vi "speed_test.vi"() -> ()   [LabVIEW 2010]
panel:
  out "XY Graph 2":cluster{i32[], dbl[]}(graph)
  out "Numeric":i32
  out "XY Graph":cluster{i32[], dbl[]}(graph)
  out "resulting string":string
  in  "spot":dbl[](array[numeric])
  # "x"
  # "y"
  # "z"
  # "I"
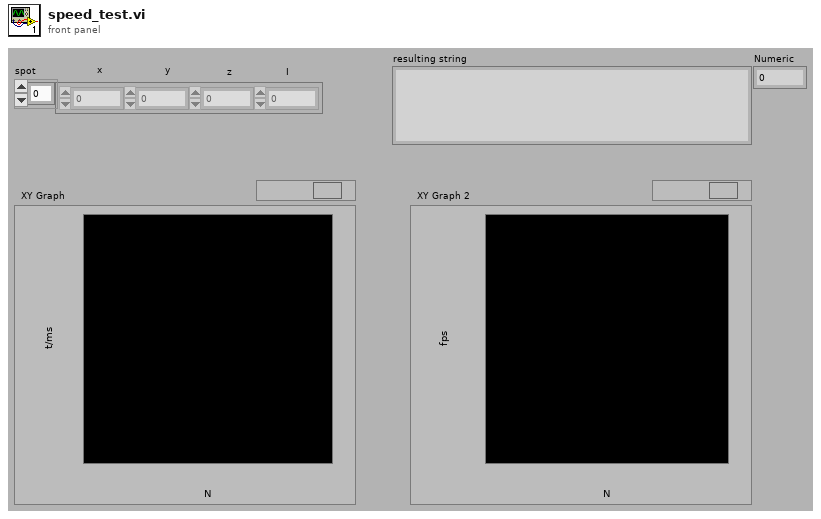
[diagram p1: front panel]
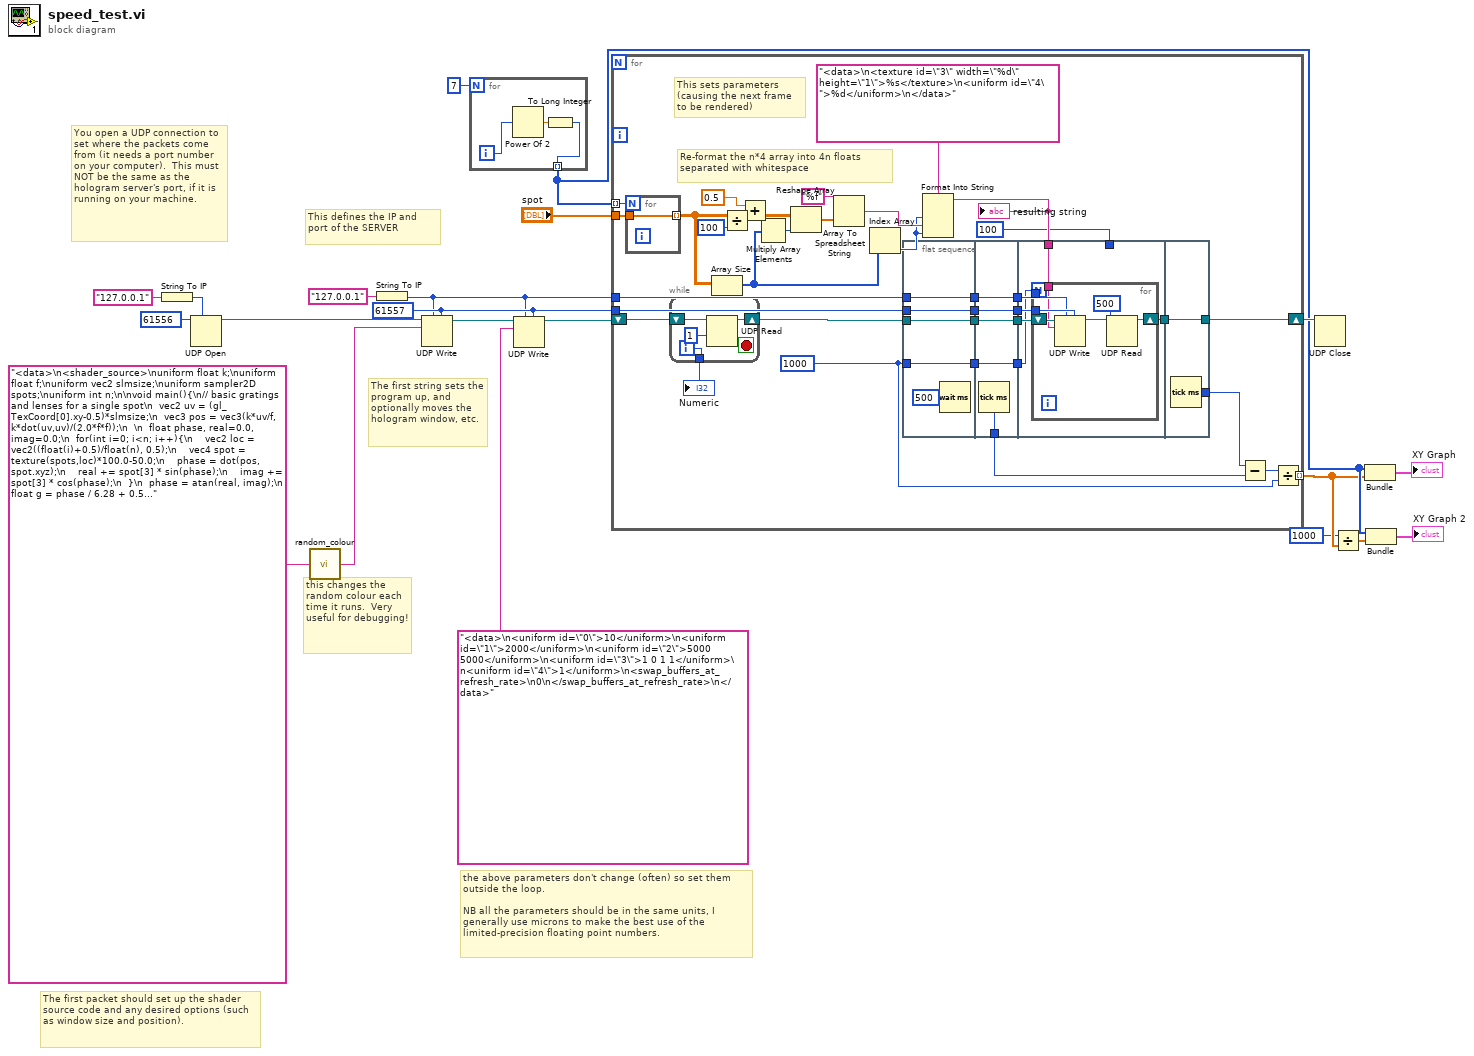
[diagram p0: block diagram]
diagram:
  w15 = u16 61557 ("port")
  # "The first packet should set up the shader source code and any desired options (such as window size and position)."
  # "This defines the IP and port of the SERVER"
  # "the above parameters don't change (often) so set them outside the loop.\n\nNB all the parameters should be in the same units, I generally use microns to make the best use of the limited-precision floating point numbers."
  # "You open a UDP connection to set where the packets come from (it needs a port number on your computer).  This must NOT be the same as the hologram server's port, if it is running on your machine."
  # "The first string sets the program up, and optionally moves the hologram window, etc."
  # "this changes the random colour each time it runs.  Very useful for debugging!"
  n1 = String To IP(1:"127.0.0.1" ("name")) -> (0:w14:u32)
  n2 = UDP Open(7:w14, 11:u16 61556 ("port")) -> (port=w21:refnum<k16>)  [unwired: 3 in, 2 out]
  n3 = call "random_colour.vi"("string in"="<data>\n<shader_source>\nuniform float k;\nuniform float f;\nuniform vec2 slmsize;\nuniform sampler2D spots;\nuniform int n;\n\nvoid main(){\n// basic gratings and lenses for a single spot\n  vec2 uv = (gl_TexCoord[0].xy-0.5)*slmsize;\n  vec3 pos = vec3(k*uv/f, k*dot(uv,uv)/(2.0*f*f));\n  \n  float phase, real=0.0, imag=0.0;\n  for(int i=0; i<n; i++){\n    vec2 loc = vec2((float(i)+0.5)/float(n), 0.5);\n    vec4 spot = texture(spots,loc)*100.0-50.0;\n    phase = dot(pos, spot.xyz);\n    real += spot[3] * sin(phase);\n    imag += spot[3] * cos(phase);\n  }\n  phase = atan(real, imag);\n  float g = phase / 6.28 + 0.5; // map -pi to pi onto zero to one\n\n  gl_FragColor=vec4(g,g,g,1.0);\n\n//  gl_FragColor = vec4(%%randcol%%);\n}\n</shader_source>\n<window_rect>\n0 0 512 512\n</window_rect>\n<network_reply>\n1\n</network_reply>\n</data> " ("data in")) -> ("string out, with %%randcol%% replaced with a 4-element colour"=w16:string)
  n4 = String To IP(1:"127.0.0.1" ("name")) -> (0:w9:u32)
  n5 = UDP Write(address=w9, port or service name=w15, connection ID=w21, data in=w16) -> (3:w12:refnum<k16>)  [unwired: 2 in, 1 out]
  n6 = for {
    N: 7 -> [_]
    tunnel: [w22] -> w4 mode=indexing
    i -> [w24]
    n7 = Power Of 2(x=w24) -> (2^x=w23:dbl)
    n8 = To Long Integer(number=w23) -> (32bit integer=w22:i32)
  }
  n9 = UDP Write(address=w9, port or service name=w15, connection ID=w12, data in="<data>\n<uniform id=\"0\">10</uniform>\n<uniform id=\"1\">2000</uniform>\n<uniform id=\"2\">5000 5000</uniform>\n<uniform id=\"3\">1 0 1 1</uniform>\n<uniform id=\"4\">1</uniform>\n<swap_buffers_at_refresh_rate>\n0\n</swap_buffers_at_refresh_rate>\n</data>") -> (3:w13:refnum<k16>)  [unwired: 2 in, 1 out]
  n10 = for {
    tunnel: w15 -> [w50]
    tunnel: w9 -> [w48]
    tunnel: [w30] -> w2 mode=indexing
    tunnel: "spot" -> [w29]
    shift-right: [w51] -> w19
    shift-left: w13 -> [w49]
    tunnel: w4 -> [w27] mode=indexing
    w31 = 1000
    # "Re-format the n*4 array into 4n floats separated with whitespace"
    # "This sets parameters\n(causing the next frame\nto be rendered)"
    n11 = for {
      N: w27 -> [_]
      tunnel: w29 -> [w66]
      tunnel: [w66] -> w28 mode=indexing
    }
    n12 = while {
      shift-right: [w64] -> w26
      shift-left: w49 -> [w65]
      tunnel: [w62] -> w25
      i -> [w62]
      stop <- w61 stop-if-true
      n13 = UDP Read(connection ID=w65, timeout ms (25000)=1) -> (error out=w61:errorcluster, 3:w64:refnum<k16>)  [unwired: 2 in, 3 out]
    }
    "Numeric" <- w25
    n14 = Array Size(array=w28) -> (size(s)=w45:i32[])
    n15 = Divide(x=w28, y=100) -> (x/y=w39:dbl[][])
    n16 = Add(x=0.5, y=w39) -> (x+y=w37:dbl[][])
    n17 = Multiply Array Elements(1:w45) -> (0:w44:i32)
    n18 = Reshape Array(w37, w44) -> (w43:dbl[])
    n19 = Array To Spreadsheet String(array=w43, 3:"%f" ("format string")) -> (spreadsheet string=w42:string)  [unwired: 1 in]
    n20 = Index Array(array=w45) -> (element=w35:i32)  [unwired: 1 in]
    n21 = flat-sequence {
      tunnel: w31 -> [w68]
      tunnel: w48 -> [w69]
      tunnel: w26 -> [w70]
      tunnel: w50 -> [w71]
      tunnel: [w71] -> w60
      tunnel: [w70] -> w59
      tunnel: [w69] -> w58
      tunnel: [w68] -> w57
      tunnel: [w76] -> w56
      tunnel: [w75] -> w55
      tunnel: [w74] -> w54
      tunnel: [w73] -> w53
      tunnel: w60 -> [w76]
      tunnel: w59 -> [w75]
      tunnel: w58 -> [w74]
      tunnel: w57 -> [w73]
      tunnel: [w72] -> w33
      tunnel: w47 -> [w78]
      tunnel: u32 100 ("millisecond multiple") -> [_]
      tunnel: w56 -> [w81]
      tunnel: w55 -> [w80]
      tunnel: w54 -> [w79]
      tunnel: w53 -> [w77]
      tunnel: [w82] -> w52
      tunnel: [w91] -> w51
      tunnel: w52 -> [w91]
      tunnel: [w90] -> w34
      frame #0 {
        n22 = Wait (ms)(milliseconds to wait=u32 500) -> ()  [unwired: 1 out]
      }
      frame #1 {
        n23 = Tick Count (ms)() -> (millisecond timer value=w72:u32)
      }
      frame #2 {
        n24 = for {
          N: w77 -> [_]
          tunnel: w81 -> [w88]
          tunnel: w79 -> [w86]
          tunnel: w78 -> [w84]
          shift-right: [w89] -> w82
          shift-left: w80 -> [w87]
          n25 = UDP Write(address=w86, port or service name=w88, connection ID=w87, data in=w84) -> (3:w85:refnum<k16>)  [unwired: 2 in, 1 out]
          n26 = UDP Read(connection ID=w85, timeout ms (25000)=500) -> (3:w89:refnum<k16>)  [unwired: 2 in, 4 out]
        }
      }
      frame #3 {
        n27 = Tick Count (ms)() -> (millisecond timer value=w90:u32)
      }
    }
    n28 = Format Into String(format string="<data>\n<texture id=\"3\" width=\"%d\" height=\"1\">%s</texture>\n<uniform id=\"4\">%d</uniform>\n</data>" ("data in"), w35, w42, w35) -> (resulting string=w47:string)  [unwired: 2 in, 1 out]
    "resulting string" <- w47
    n29 = Subtract(x=w34, y=w33) -> (x-y=w32:u32)
    n30 = Divide(x=w32, y=w31) -> (x/y=w30:dbl)
  }
  n31 = UDP Close(connection ID=w19) -> ()  [unwired: 1 in, 2 out]
  n32 = Divide(x=1000, y=w2) -> (x/y=w3:dbl[])
  n33 = Bundle(w4, w2) -> (→"XY Graph":cluster{i32[], dbl[]})  [unwired: 1 in]
  n34 = Bundle(w4, w3) -> (→"XY Graph 2":cluster{i32[], dbl[]})  [unwired: 1 in]
